vi "XW_Type_1a_correction.vi"(1 "Tmeas (degC)":dbl, 2 "Calib consts.":dbl[](array[numeric])) -> (0 "Corrected calib consts.":dbl[](array[numeric]))   [LabVIEW 2010]
panel:
  # "Type 1a: Open ended. Single calibration corrected to conditions at t"
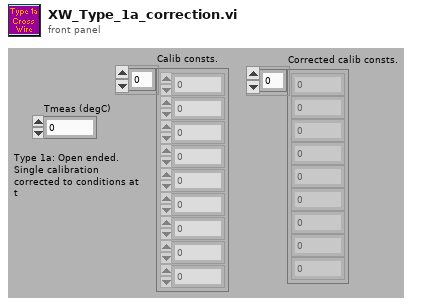
[diagram p1: front panel]
types:
  T1 = cluster{"Calib consts.[0]":dbl, "Calib consts.[1]":dbl, "Calib consts.[2]":dbl, "Calib consts.[3]":dbl, "Calib consts.[4]":dbl, "Calib consts.[5]":dbl, "Calib consts.[6]":dbl, "Calib consts.[7]":dbl, "Calib consts.[8]":dbl, "Calib consts.[9]":dbl, "Calib consts.[10]":dbl, "Calib consts.[11]":dbl, "Calib consts.[12]":dbl, "Calib consts.[13]":dbl, "Calib consts.[14]":dbl, "Calib consts.[15]":dbl, "Calib consts.[16]":dbl, "Calib consts.[17]":dbl}
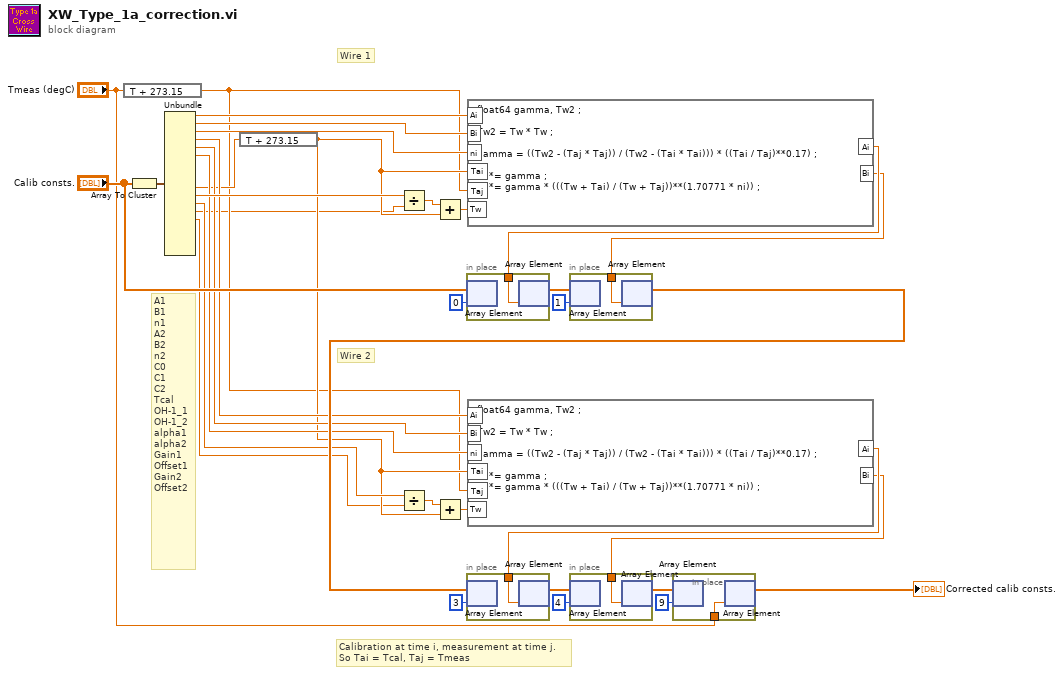
[diagram p0: block diagram]
diagram:
  # "Calibration at time i, measurement at time j.\nSo Tai = Tcal, Taj = Tmeas"
  # "Wire 1"
  # "Wire 2"
  # "A1\nB1\nn1\nA2\nB2\nn2\nC0\nC1\nC2\nTcal\nOH-1_1\nOH-1_2\nalpha1\nalpha2\nGain1\nOffset1\nGain2\nOffset2"
  n1 = expression code="T + 273.15"("Tmeas (degC)") -> (w20:dbl)
  n2 = Array To Cluster(array="Calib consts.") -> (cluster=w34:T1)
  n3 = Unbundle(w34) -> ("Calib consts.[0]"=w33:dbl, "Calib consts.[1]"=w32:dbl, "Calib consts.[2]"=w31:dbl, "Calib consts.[3]"=w23:dbl, "Calib consts.[4]"=w24:dbl, "Calib consts.[5]"=w25:dbl, "Calib consts.[9]"=w22:dbl, "Calib consts.[10]"=w27:dbl, "Calib consts.[11]"=w26:dbl, "Calib consts.[12]"=w2:dbl, "Calib consts.[13]"=w1:dbl)  [unwired: 7 out]
  n4 = expression code="T + 273.15"(w22) -> (w21:dbl)
  n5 = Divide(x=w27, y=w2) -> (x/y=w18:dbl)
  n6 = Divide(x=w26, y=w1) -> (x/y=w11:dbl)
  n7 = Add(x=w18, y=w21) -> (x+y=w17:dbl)
  n8 = Add(x=w11, y=w21) -> (x+y=w10:dbl)
  n9 = formula code="float64 gamma, Tw2 ;\n\nTw2 = Tw * Tw ;\n\ngamma = ((Tw2 - (Taj * Taj)) / (Tw2 - (Tai * Tai))) * ((Tai / Taj)**0.17) ;\n\nAi *= gamma ;\nBi *= gamma * (((Tw + Tai) / (Tw + Taj))**(1.70771 * ni)) ;"("Ai"=w33, "Bi"=w32, "ni"=w31, "Tai"=w21, "Taj"=w20, "Tw"=w17) -> ("Ai"=w15:dbl, "Bi"=w14:dbl)
  n10 = in-place {
    in-place-border: w15 -> [w35]
    n11 = in-place-array #1("Calib consts.", 0) -> ()  [unwired: 1 out]
    n12 = in-place-array #1(w35) -> (w12:dbl[])  [unwired: 1 out]
  }
  n13 = formula code="float64 gamma, Tw2 ;\n\nTw2 = Tw * Tw ;\n\ngamma = ((Tw2 - (Taj * Taj)) / (Tw2 - (Tai * Tai))) * ((Tai / Taj)**0.17) ;\n\nAi *= gamma ;\nBi *= gamma * (((Tw + Tai) / (Tw + Taj))**(1.70771 * ni)) ;"("Ai"=w23, "Bi"=w24, "ni"=w25, "Tai"=w21, "Taj"=w20, "Tw"=w10) -> ("Ai"=w8:dbl, "Bi"=w7:dbl)
  n14 = in-place {
    in-place-border: w14 -> [w36]
    n15 = in-place-array #2(w12, 1) -> ()  [unwired: 1 out]
    n16 = in-place-array #2(w36) -> (w29:dbl[])  [unwired: 1 out]
  }
  n17 = in-place {
    in-place-border: w8 -> [w37]
    n18 = in-place-array #3(w29, 3) -> ()  [unwired: 1 out]
    n19 = in-place-array #3(w37) -> (w5:dbl[])  [unwired: 1 out]
  }
  n20 = in-place {
    in-place-border: w7 -> [w38]
    n21 = in-place-array #4(w5, 4) -> ()  [unwired: 1 out]
    n22 = in-place-array #4(w38) -> (w3:dbl[])  [unwired: 1 out]
  }
  n23 = in-place {
    in-place-border: "Tmeas (degC)" -> [w39]
    n24 = in-place-array #5(w3, 9) -> ()  [unwired: 1 out]
    n25 = in-place-array #5(w39) -> (→"Corrected calib consts.":dbl[])  [unwired: 1 out]
  }
